vi "getChannel.vi"(8 "error in (no error)":errorcluster, 9 "Channel":u16, 11 "Instrument.Amplifier in":refnum<class "Instrument.Amplifier.lvclass">) -> (0 "error out":errorcluster, 2 "channelProperties":variant, 3 "Instrument.Amplifier out":refnum<class "Instrument.Amplifier.lvclass">)   [LabVIEW 2019, in "Instrument.Amplifier.lvclass"]
uses:
  Instrument.Amplifier.lvclass
  Amplifier.Commands--Enum.ctl
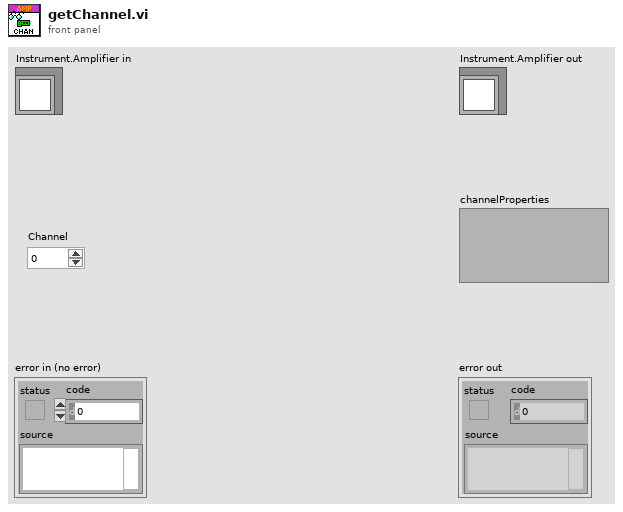
[diagram p1: front panel]
types:
  T1 = typedef "Instrument.Amplifier.lvclass/Amplifier.Commands--Enum.ctl" = enum16{"getChannel", "getAllChannels", "setChannel", "setAllChannels"}
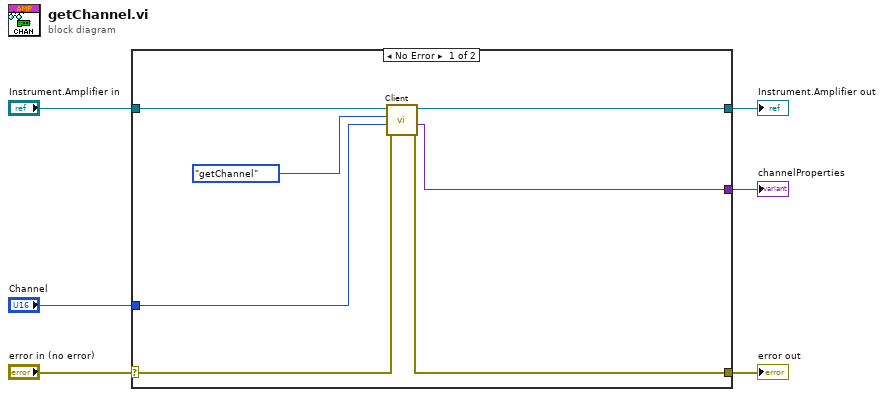
[diagram p0: block diagram]
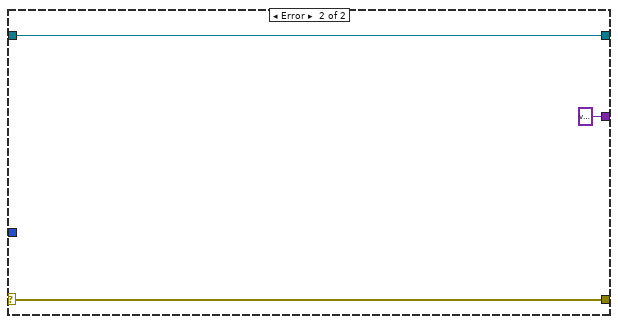
[diagram p2: hidden frame]
diagram:
  n1 = case shown="No Error" "error in (no error)" {
    selector: "error in (no error)" -> [w11 w16]
    tunnel: [w9 w16] -> w5
    tunnel: [w13 w15] -> w3
    tunnel: "Instrument.Amplifier in" -> [w7 w15]
    tunnel: [w10 variant ("Data out")] -> w2
    tunnel: "Channel" -> [w12 _]
    frame No Error {
      n2 = call-dynamic "Client.vi"("error in (no error)"=w11, "Data in"=w12, "Command in"=Amplifier.Commands--Enum."getChannel" ("Commands"), "Instrument in"=w7) -> ("error out"=w9:errorcluster, "Data out"=w10:variant, "Instrument out"=w13:refnum<class "Instrument.Amplifier.lvclass">)  [unwired: 4 in, 1 out]
    }
    frame Error {
    }
  }
  "error out" <- w5
  "Instrument.Amplifier out" <- w3
  "channelProperties" <- w2
